vi "CompileParseAWGPulse.vi"(0 "RF Array":variant[](array[variant])) -> (1 "MWout":T1[](array[typedef]), 2 "RFout":T1[](array[typedef]))   [LabVIEW 2019]
uses:
  controls/AWGpulse.ctl
  controls/AWGchannelcontrol.ctl
panel:
  in  "Array 4":T1[](array[typedef])=[{"Name"="PREP: Cooling", "time det"=6500.0, "time step"=0.0, "Channel Array"=[{"freq\n"=113002.236, "freq step"=0.0, "amp det"=50.0, "amp step"=0.0, "phase det"=0.0, "phase step"=0.0}, {"freq\n"=87024.063, "freq step"=0.0, "amp det"=50.0, "amp step"=0.0, "phase det"=0.0, "phase step"=0.0}, {"freq\n"=109792.759, "freq step"=0.0, "amp det"=50.0, "amp step"=0.0, "phase det"=0.0, "phase step"=0.0}, {"freq\n"=90222.036, "freq step"=0.0, "amp det"=50.0, "amp step"=0.0, "phase det"=0.0, "phase step"=0.0}]}, {"Name"="RF padding", "time det"=6500.0, "time step"=0.0, "Channel Array"=[{"freq\n"=0.0, "freq step"=0.0, "amp det"=0.0, "amp step"=0.0, "phase det"=0.0, "phase step"=0.0}]}, {"Name"="MW Padding", "time det"=40.0, "time step"=0.0, "Channel Array"=[{"freq\n"=0.0, "freq step"=0.0, "amp det"=0.0, "amp step"=0.0, "phase det"=0.0, "phase step"=0.0}]}, {"Name"="RF Padding", "time det"=40.0, "time step"=0.0, "Channel Array"=[{"freq\n"=0.0, "freq step"=0.0, "amp det"=0.0, "amp step"=0.0, "phase det"=0.0, "phase step"=0.0}]}, {"Name"="MW Padding", "time det"=800.0, "time step"=0.0, "Channel Array"=[{"freq\n"=0.0, "freq step"=0.0, "amp det"=0.0, "amp step"=0.0, "phase det"=0.0, "phase step"=0.0}]}, {"Name"="RF Padding", "time det"=800.0, "time step"=0.0, "Channel Array"=[{"freq\n"=0.0, "freq step"=0.0, "amp det"=0.0, "amp step"=0.0, "phase det"=0.0, "phase step"=0.0}]}, {"Name"="PREP: Cooling", "time det"=6500.0, "time step"=0.0, "Channel Array"=[{"freq\n"=113002.236, "freq step"=0.0, "amp det"=50.0, "amp step"=0.0, "phase det"=0.0, "phase step"=0.0}, {"freq\n"=87024.063, "freq step"=0.0, "amp det"=50.0, "amp step"=0.0, "phase det"=0.0, "phase step"=0.0}, {"freq\n"=109792.759, "freq step"=0.0, "amp det"=50.0, "amp step"=0.0, "phase det"=0.0, "phase step"=0.0}, {"freq\n"=90222.036, "freq step"=0.0, "amp det"=50.0, "amp step"=0.0, "phase det"=0.0, "phase step"=0.0}]}, {"Name"="RF padding", "time det"=6500.0, "time step"=0.0, "Channel Array"=[{"freq\n"=0.0, "freq step"=0.0, "amp det"=0.0, "amp step"=0.0, "phase det"=0.0, "phase step"=0.0}]}, {"Name"="MW Padding", "time det"=40.0, "time step"=0.0, "Channel Array"=[{"freq\n"=0.0, "freq step"=0.0, "amp det"=0.0, "amp step"=0.0, "phase det"=0.0, "phase step"=0.0}]}, {"Name"="RF Padding", "time det"=40.0, "time step"=0.0, "Channel Array"=[{"freq\n"=0.0, "freq step"=0.0, "amp det"=0.0, "amp step"=0.0, "phase det"=0.0, "phase step"=0.0}]}, {"Name"="Freq scan clock1", "time det"=984.2, "time step"=0.0, "Channel Array"=[{"freq\n"=100013.993, "freq step"=0.1, "amp det"=17.0, "amp step"=0.0, "phase det"=0.0, "phase step"=1.0}]}, {"Name"="MW Padding", "time det"=800.0, "time step"=0.0, "Channel Array"=[{"freq\n"=0.0, "freq step"=0.0, "amp det"=0.0, "amp step"=0.0, "phase det"=0.0, "phase step"=0.0}]}, {"Name"="RF Padding", "time det"=800.0, "time step"=0.0, "Channel Array"=[{"freq\n"=0.0, "freq step"=0.0, "amp det"=0.0, "amp step"=0.0, "phase det"=0.0, "phase step"=0.0}]}, {"Name"="Line trig set", "time det"=10.0, "time step"=0.0, "Channel Array"=[{"freq\n"=113002.236, "freq step"=0.0, "amp det"=50.0, "amp step"=0.0, "phase det"=0.0, "phase step"=0.0}, {"freq\n"=87024.063, "freq step"=0.0, "amp det"=50.0, "amp step"=0.0, "phase det"=0.0, "phase step"=0.0}, {"freq\n"=109792.759, "freq step"=0.0, "amp det"=50.0, "amp step"=0.0, "phase det"=0.0, "phase step"=0.0}, {"freq\n"=90222.036, "freq step"=0.0, "amp det"=50.0, "amp step"=0.0, "phase det"=0.0, "phase step"=0.0}]}, {"Name"="RF padding", "time det"=10.0, "time step"=0.0, "Channel Array"=[{"freq\n"=0.0, "freq step"=0.0, "amp det"=0.0, "amp step"=0.0, "phase det"=0.0, "phase step"=0.0}]}]
  out "Array":T3(array[cluster])
  in  "error in":errorcluster
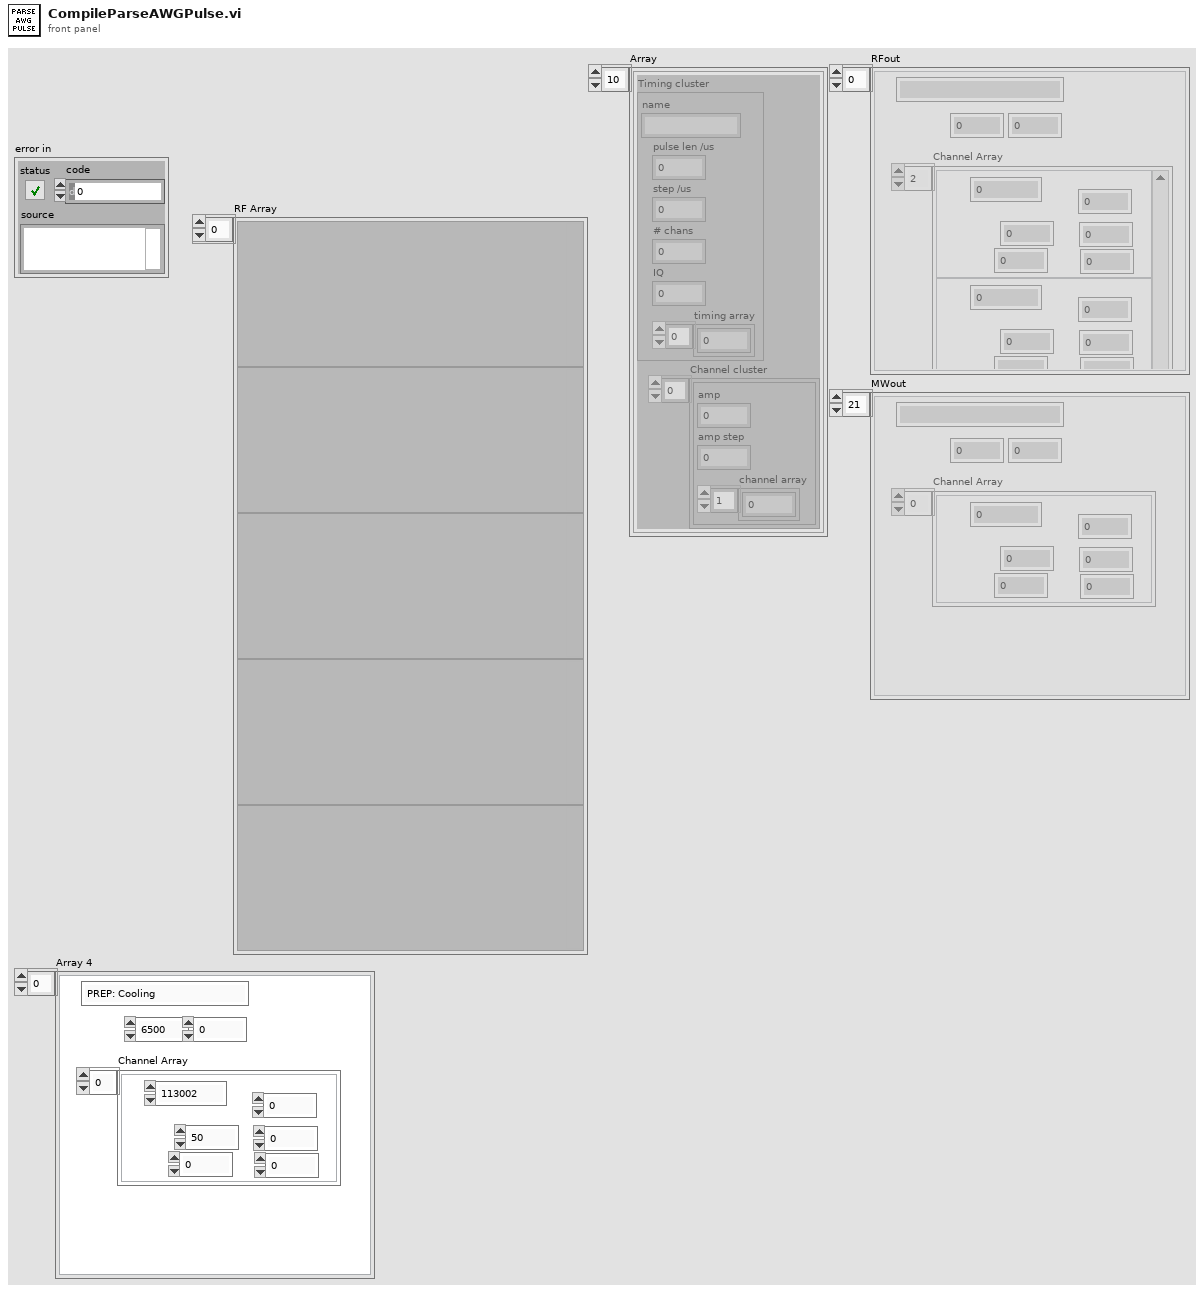
[diagram p1: front panel]
types:
  T1 = typedef "AWGpulse.ctl" = cluster{"Name":string, "time det":dbl, "time step":dbl, "Channel Array":T2[]}
  T2 = typedef "AWGchannelcontrol.ctl" = cluster{"freq\n":dbl, "freq step":dbl, "amp det":dbl, "amp step":dbl, "phase det":dbl, "phase step":dbl}
  T3 = cluster{"Timing cluster":cluster{"name":string, "pulse len /us":dbl, "step /us":dbl, "# chans":i32, "IQ":i32, "timing array":dbl[]}, "Channel cluster":cluster{"amp":dbl, "amp step":dbl, "channel array":dbl[]}[]}[]
  T4 = cluster{"Timing cluster":cluster{"name":string, "pulse len /us":dbl, "step /us":dbl, "# chans":i32, "IQ":i32, "timing array":dbl[]}, "Channel cluster":cluster{"amp":dbl, "amp step":dbl, "channel array":dbl[]}[]}
  T5 = cluster{"name":string, "pulse len /us":dbl, "step /us":dbl, "# chans":i32, "IQ":i32, "timing array":dbl[]}
  T6 = cluster{"amp":dbl, "amp step":dbl, "channel array":dbl[]}[]
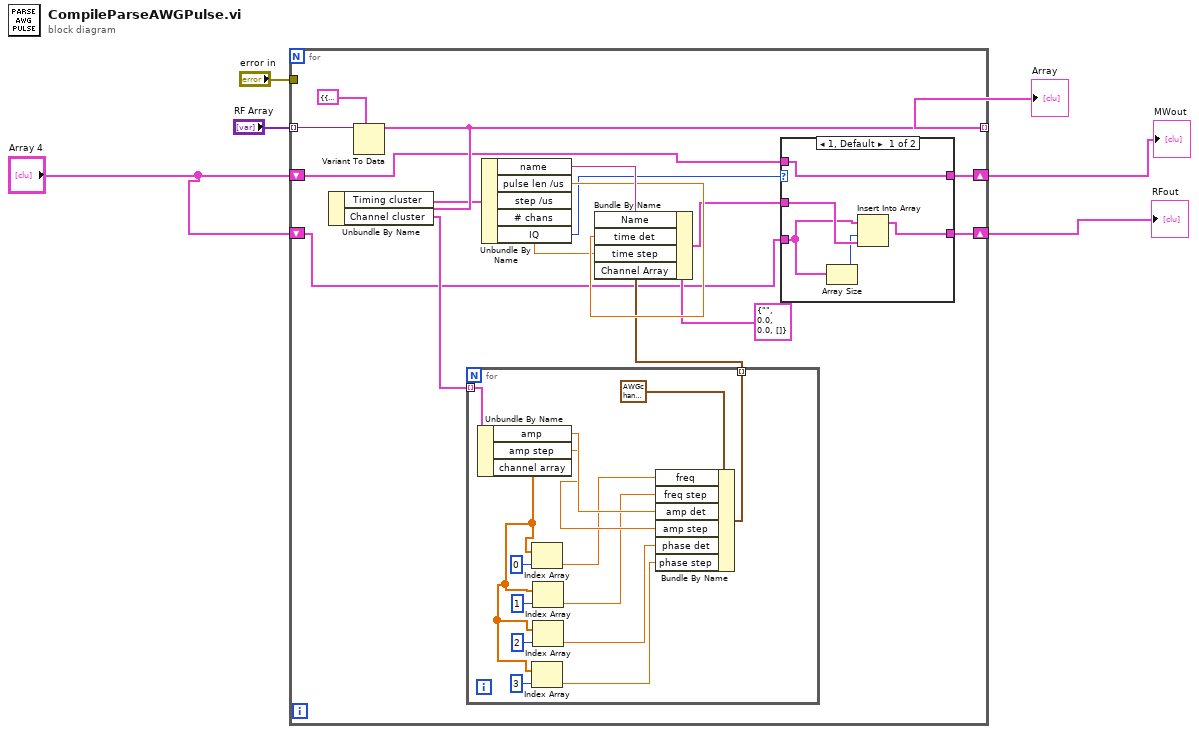
[diagram p0: block diagram]
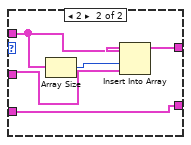
[diagram p2: hidden frame]
diagram:
  n1 = for {
    tunnel: "RF Array" -> [w21] mode=indexing
    tunnel: "error in" -> [_]
    tunnel: [w20] -> w4 mode=indexing
    shift-right: [w8] -> w2
    shift-left: "Array 4" -> [w10]
    shift-right: [w7] -> w3
    shift-left: "Array 4" -> [w9]
    n2 = Variant To Data(type=T4 {"Timing cluster"={"name"="RF padding", "pulse len /us"=10.0, "step /us"=0.0, "# chans"=1, "IQ"=1, "timing array"=[0.0]}, "Channel cluster"=[{"amp"=0.0, "amp step"=0.0, "channel array"=[0.0, 0.0, 0.0, 0.0]}]} ("output cluster"), Variant=w21) -> (data=w20:T4)  [unwired: 1 in, 1 out]
    n3 = Unbundle By Name(w20) -> ("Timing cluster"=w19:T5, "Channel cluster"=w14:T6)
    n4 = for {
      tunnel: w14 -> [w45] mode=indexing
      tunnel: [w33] -> w13 mode=indexing
      n5 = Unbundle By Name(w45) -> ("amp"=w44:dbl, "amp step"=w43:dbl, "channel array"=w35:dbl[])
      n6 = Index Array(array=w35, index=0) -> (element=w41:dbl)
      n7 = Index Array(array=w35, index=3) -> (element=w37:dbl)
      n8 = Index Array(array=w35, index=1) -> (element=w39:dbl)
      n9 = Index Array(array=w35, index=2) -> (element=w34:dbl)
      n10 = Bundle By Name(cluster=T2 {"freq\n"=0.0, "freq step"=0.0, "amp det"=0.0, "amp step"=0.0, "phase det"=0.0, "phase step"=0.0} ("ChannelCluster"), "freq"=w41, "freq step"=w39, "amp det"=w44, "amp step"=w43, "phase det"=w34, "phase step"=w37) -> (w33:T2)
    }
    n11 = Unbundle By Name(w19) -> ("name"=w18:string, "pulse len /us"=w17:dbl, "step /us"=w16:dbl, "IQ"=w12:i32)  [unwired: 1 out]
    n12 = Bundle By Name(cluster=T1 {"Name"="", "time det"=0.0, "time step"=0.0, "Channel Array"=[]} ("AWGPulseCluster"), "Name"=w18, "time det"=w17, "time step"=w16, "Channel Array"=w13) -> (w11:T1)
    n13 = case shown="1, Default" w12 {
      tunnel: w11 -> [w25 w31]
      tunnel: w10 -> [w27 w29]
      tunnel: w9 -> [w24 w32]
      tunnel: [w27 w30] -> w8
      tunnel: [w26 w32] -> w7
      frame 1, Default {
        n14 = Array Size(array=w24) -> (size(s)=w23:i32)
        n15 = Insert Into Array(array=w24, index=w23, new element=w25) -> (w26:T1[])
      }
      frame 2 {
        n16 = Array Size(array=w29) -> (size(s)=w28:i32)
        n17 = Insert Into Array(array=w29, index=w28, new element=w31) -> (w30:T1[])
      }
    }
  }
  "Array" <- w4
  "RFout" <- w3
  "MWout" <- w2
